vi "Number To Percent.vi"(1 "Array In":cluster{"Label":string, "Value":dbl}[](array[cluster])) -> (0 "Array Out":cluster{"Label":string, "Value":dbl}[](array[cluster]))   [LabVIEW 2016, in "CML UI.lvlib" / "Circular Cue Helper.lvlib"]
uses:
  Circular Cue Helper.lvlib
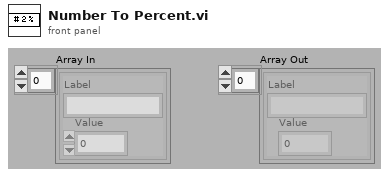
[diagram p1: front panel]
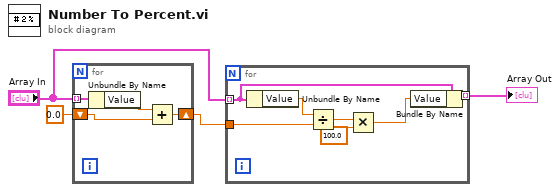
[diagram p0: block diagram]
diagram:
  n1 = for {
    tunnel: "Array In" -> [w8] mode=indexing
    shift-right: [w6] -> w3
    shift-left: 0.0 -> [w5]
    n2 = Unbundle By Name(w8) -> ("Value"=w7:dbl)
    n3 = Add(x=w7, y=w5) -> (x+y=w6:dbl)
  }
  n4 = for {
    tunnel: "Array In" -> [w13] mode=indexing
    tunnel: w3 -> [w14]
    tunnel: [w10] -> w4 mode=indexing
    n5 = Unbundle By Name(w13) -> ("Value"=w15:dbl)
    n6 = Divide(x=w15, y=w14) -> (x/y=w12:dbl)
    n7 = Multiply(x=w12, y=100.0) -> (x*y=w9:dbl)
    n8 = Bundle By Name(cluster=w13, "Value"=w9) -> (w10:cluster{"Label":string, "Value":dbl})
  }
  "Array Out" <- w4
